vi "Disable MPG.vi"(8 "error in":errorcluster, 11 "Gantry in":refnum<class "Gantry.lvclass">) -> (0 "error out":errorcluster, 3 "Gantry out":refnum<class "Gantry.lvclass">)   [LabVIEW 2026, in "Gantry.lvclass"]
uses:
  Gantry.lvclass
  <instrlib>/Aerotech Automation1/Aerotech Automation1.lvlib
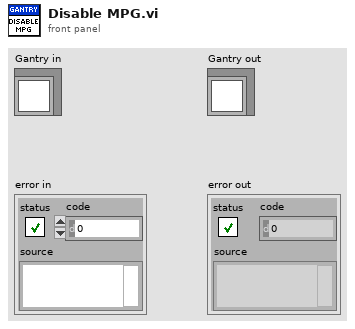
[diagram p1: front panel]
types:
  T1 = typedef "Virtual Modes.ctl" = enum16{"Nonvirtual", "Virtual"}
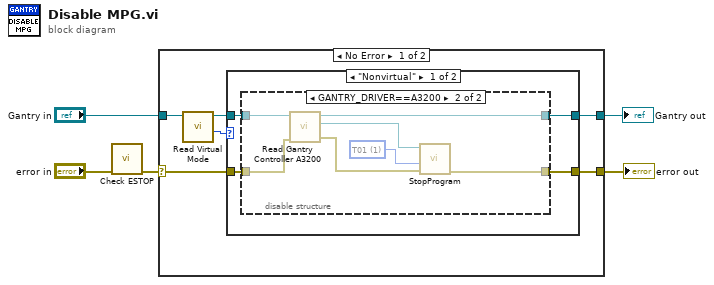
[diagram p0: block diagram]
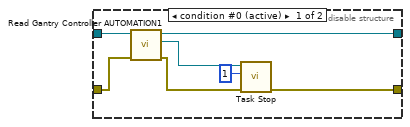
[diagram p2: hidden frame]
diagram:
  n1 = call "Check ESTOP.vi"("error in"="error in") -> ("error out"=w2:errorcluster)  [unwired: 10 in]
  n2 = case shown="No Error" w2 {
    selector: w2 -> [w10 w33]
    tunnel: [w9 w33] -> w5
    tunnel: [w11 w32] -> w4
    tunnel: "Gantry in" -> [w8 w32]
    frame No Error {
      n3 = call-dynamic "Read Virtual Mode.vi"("Gantry in"=w8) -> ("Virtual Mode"=w6:T1, "Gantry out"=w7:refnum<class "Gantry.lvclass">)  [unwired: 7 in, 2 out]
      n4 = case shown="\"Nonvirtual\"" w6 {
        tunnel: [w13 w31] -> w11
        tunnel: w10 -> [w14 w30]
        tunnel: [w12 w30] -> w9
        tunnel: w7 -> [w15 w31]
        frame "Nonvirtual" {
          n5 = disable-structure shown="GANTRY_DRIVER==A3200" {
            disable-tunnel: w15 -> [w22 w26]
            disable-tunnel: w14 -> [w21 w25]
            disable-tunnel: [w20 w24] -> w13
            disable-tunnel: [w17 w23] -> w12
            frame condition #0 (active) {
              n6 = call "Read Gantry Controller AUTOMATION1.vi"("error in (no error)"=w21, "Gantry in"=w22) -> ("error out"=w18:errorcluster, "Controller AUTOMATION1"=w19:refnum<k24>, "Gantry out"=w20:refnum<class "Gantry.lvclass">)  [unwired: 7 in]
              n7 = call <instrlib>:"Task Stop.vi"("error in (no error)"=w18, "Task Index"=1, "Controller Refnum"=w19) -> ("error out"=w17:errorcluster)  [unwired: 7 in, 1 out]
            }
            frame condition #1 {
              w29 = 1 items=["TLibrary", "T01", "T02", "T03", "T04", "T05", "T06", "T07", "T08", "T09", "T10", "T11", "T12", "T13", "T14", "T15", "T16", "T17", "T18", "T19", "T20", "T21", "T22", "T23", "T24", "T25", "T26", "T27", "T28", "T29", "T30", "T31"] ("taskId")
              n8 = call "Read Gantry Controller A3200.vi"("error in (no error)"=w25, "Gantry in"=w26) -> ("error out"=w28:errorcluster, "A3200 controller out"=w27:refnum<k24>, "Gantry out"=w24:refnum<class "Gantry.lvclass">)  [unwired: 7 in]
              n9 = call "StopProgram.vi"("error in (no error)"=w28, "taskId"=w29, "controller in"=w27) -> ("error out"=w23:errorcluster)  [unwired: 7 in, 1 out]
            }
          }
        }
        frame "Virtual" {
        }
      }
    }
    frame Error {
    }
  }
  "error out" <- w5
  "Gantry out" <- w4
